vi "Get driving mode to excecute.vi"() -> (0 "Drive Mode":T1=enum."Driver Operated")   [LabVIEW 2018]
uses:
  Drive mode.ctl
  Robot Global Data.vi
  <vilib>/Rock Robotics/Network Tables/NT Read Boolean.vi
panel:
  # "Choose which mode to excecute"
  # "IDK HOw this is going to work exactly"
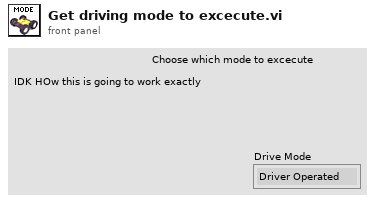
[diagram p1: front panel]
types:
  T1 = typedef "Drive mode.ctl" = enum16{"HAB2toHAB1", "Driver Operated", "Drive Autonomously", "Disabled"}
  T2 = typedef "WPI_DriverStationRobotMode2.ctl" = enum16{"Autonomous Disabled", "Autonomous Enabled", "Teleop Disabled", "Teleop Enabled", "Disconnected", "Finish", "Test Disabled", "Test Enabled", "Emergency Stopped"}
  T3 = cluster{"Left Motor Value":dbl, "Right Motor Value":dbl}
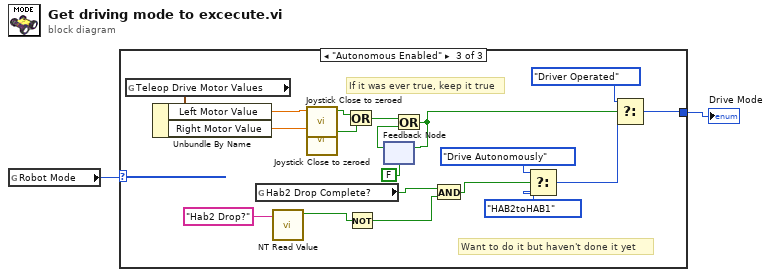
[diagram p0: block diagram]
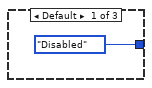
[diagram p2: hidden frame]
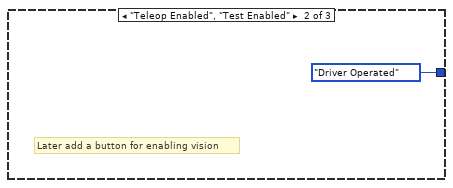
[diagram p3: hidden frame]
diagram:
  n1 = global read "Robot Global Data.vi" "Robot Mode"() -> (w2:T2)
  n2 = case shown="\"Autonomous Enabled\"" w2 {
    tunnel: [Drive_mode."Disabled" ("Drive Mode") Drive_mode."Driver Operated" ("Drive Mode") w18] -> w1
    frame Default {
    }
    frame "Teleop Enabled", "Test Enabled" {
      # "Later add a button for enabling vision"
    }
    frame "Autonomous Enabled" {
      # "If it was ever true, keep it true"
      # "Want to do it but haven't done it yet"
      n3 = global read "Robot Global Data.vi" "Teleop Drive Motor Values"() -> (w19:T3)
      n4 = Unbundle By Name(w19) -> ("Left Motor Value"=w20:dbl, "Right Motor Value"=w21:dbl)
      n5 = global read "Robot Global Data.vi" "Hab2 Drop Complete?"() -> (w8:bool)
      n6 = call-poly <vilib>:"NT Read Value.vi"("Name"="Hab2 Drop?") -> ("Boolean"=w6:bool)  [unwired: 9 in, 1 out]
      n7 = call "Joystick Close to zeroed.vi"("Joystick"=w20) -> ("=0?"=w23:bool)  [unwired: 10 in]
      n8 = call "Joystick Close to zeroed.vi"("Joystick"=w21) -> ("=0?"=w22:bool)  [unwired: 10 in]
      n9 = Or(x=w23, y=w22) -> (x .or. y?=w14:bool)
      n10 = Not(x=w6) -> (.not. x?=w5:bool)
      n11 = feedback #1(FALSE) -> (w15:bool)
      n12 = Or(x=w14, y=w15) -> (x .or. y?=w16:bool)
      n13 = feedback-in #1(w16) -> ()
      n14 = And(x=w8, y=w5) -> (x .and. y?=w9:bool)
      n15 = Select(t=Drive_mode."Drive Autonomously" ("Drive Mode"), s=w9, f=Drive_mode."HAB2toHAB1" ("Drive Mode")) -> (s? t:f=w11:T1)
      n16 = Select(t=Drive_mode."Driver Operated" ("Drive Mode"), s=w16, f=w11) -> (s? t:f=w18:T1)
    }
  }
  "Drive Mode" <- w1
